vi "Th2829NX_PAGE_TSD.vi"() -> ()   [LabVIEW 2018]
uses:
  <vilib>/Instr/_visa.llb/VISA Configure Serial Port (Instr).vi
panel:
  out "VISA资源名称输出 2":refnum<visa-resource-name>
  in  "VISA资源名称输出":refnum<visa-resource-name>
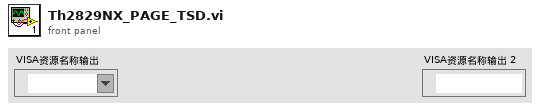
[diagram p1: front panel]
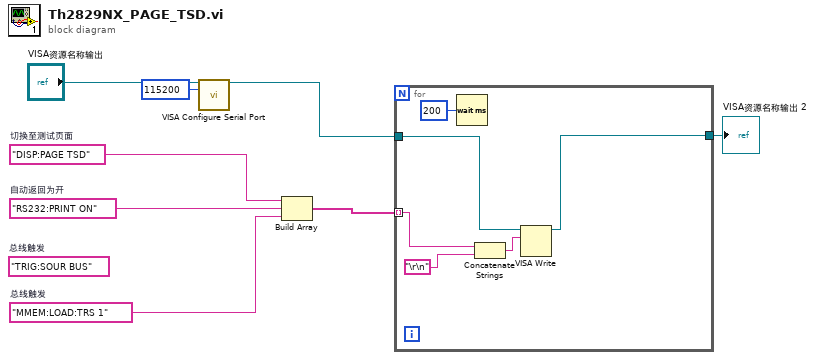
[diagram p0: block diagram]
diagram:
  w6 = "MMEM:LOAD:TRS 1"  # 总线触发
  (unwired) "TRIG:SOUR BUS"  # 总线触发
  w7 = "RS232:PRINT ON"  # 自动返回为开
  w8 = "DISP:PAGE TSD"  # 切换至测试页面
  n1 = call-poly "VISA Configure Serial Port"("VISA resource name"="VISA资源名称输出", "baud rate (9600)"=u32 115200) -> ("VISA resource name out"=w2:refnum<visa-resource-name>)  [unwired: 12 in, 1 out]
  n2 = Build Array(w8, w7, w6) -> (w5:string[])
  n3 = for {
    tunnel: w5 -> [w11] mode=indexing
    tunnel: w2 -> [w14]
    tunnel: [w12] -> w3
    n4 = Wait (ms)(milliseconds to wait=u32 200 ("等待时间（毫秒）")) -> ()  [unwired: 1 out]
    n5 = Concatenate Strings(w11, "\r\n") -> (w10:string)
    n6 = VISA Write(VISA resource name=w14, write buffer=w10) -> (VISA resource name out=w12:refnum<visa-resource-name>)  [unwired: 1 in, 2 out]
  }
  "VISA资源名称输出 2" <- w3
